vi "Update Method Event Unbundlers.vi"(8 "error in (no error)":errorcluster, 11 "VI ref in":refnum<vi>) -> (0 "error out":errorcluster, 2 "RPC Method Name":string, 3 "VI ref out":refnum<vi>)   [LabVIEW 2019, in "gRPC Scripting Tools.lvlib"]
uses:
  gRPC Scripting Tools.lvlib
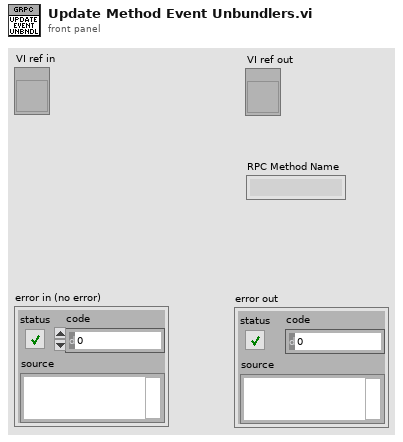
[diagram p1: front panel]
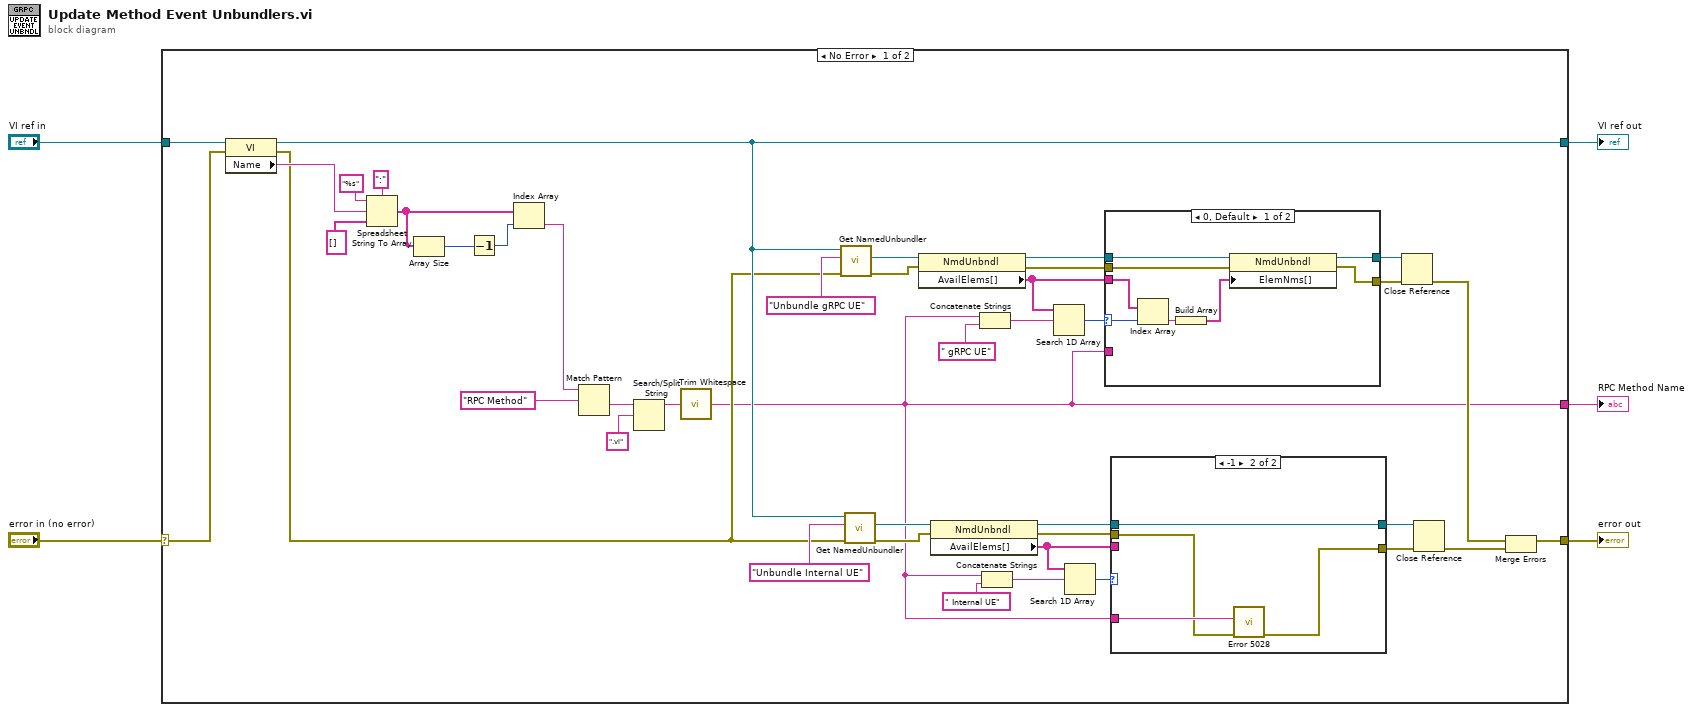
[diagram p0: block diagram]
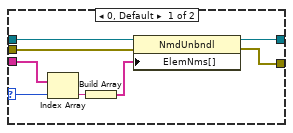
[diagram p2: hidden frame]
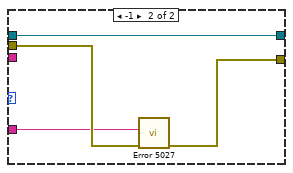
[diagram p3: hidden frame]
diagram:
  n1 = case shown="No Error" "error in (no error)" {
    selector: "error in (no error)" -> [w18 w73]
    tunnel: [w47 w73] -> w5
    tunnel: "VI ref in" -> [w29 w72]
    tunnel: [w28 w72] -> w2
    tunnel: [w6 _] -> w1
    frame No Error {
      n2 = property class="VI"(reference=w29, error in=w18) -> (reference out=w28:refnum<vi>, error out=w17:errorcluster, "Name"=w26:string)
      n3 = Spreadsheet String To Array(delimiter (Tab)=":", format string="%s", spreadsheet string=w26, array type (2D Dbl)=string[] []) -> (array=w21:string[])
      n4 = Array Size(array=w21) -> (size(s)=w23:i32)
      n5 = Decrement(x=w23) -> (x-1=w22:i32)
      n6 = Index Array(array=w21, index=w22) -> (element=w20:string)
      n7 = Match Pattern(string=w20, regular expression="RPC Method") -> (after substring=w16:string)  [unwired: 1 in, 3 out]
      n8 = Search/Split String(string=w16, search string/char (-)=".vi" ("regular expression")) -> (substring before match=w15:string)  [unwired: 1 in, 2 out]
      n9 = call <vilib>:"Trim Whitespace.vi"("string"=w15) -> ("trimmed string"=w6:string)  [unwired: 1 in]
      n10 = call "Get NamedUnbundler.vi"("error in (no error)"=w17, "Label"="Unbundle gRPC UE" ("name/order"), "Owner VI in"=w28) -> ("error out"=w43:errorcluster, "NamedUnbundler ref out"=w31:refnum<vi>)  [unwired: 5 in, 2 out]
      n11 = call "Get NamedUnbundler.vi"("error in (no error)"=w17, "Label"="Unbundle Internal UE" ("name/order"), "Owner VI in"=w28) -> ("error out"=w44:errorcluster, "NamedUnbundler ref out"=w38:refnum<vi>)  [unwired: 5 in, 2 out]
      n12 = property class="NmdUnbndl"(reference=w31, error in=w43) -> (reference out=w35:refnum<vi>, error out=w36:errorcluster, "AvailElems[]"=w34:string[])
      n13 = property class="NmdUnbndl"(reference=w38, error in=w44) -> (reference out=w12:refnum<vi>, error out=w7:errorcluster, "AvailElems[]"=w8:string[])
      n14 = Concatenate Strings(w6, " gRPC UE" ("string")) -> (w33:string)
      n15 = Concatenate Strings(w6, " Internal UE" ("string")) -> (w40:string)
      n16 = Search 1D Array(1D array=w34, element=w33) -> (index of element=w13:i32)  [unwired: 1 in]
      n17 = Search 1D Array(1D array=w8, element=w40) -> (index of element=w11:i32)  [unwired: 1 in]
      n18 = case shown="0, Default" w13 {
        selector: w13 -> [w60 _]
        tunnel: [w67 w71] -> w42
        tunnel: [w66 w69] -> w41
        tunnel: w36 -> [w65 w70]
        tunnel: w35 -> [w62 w71]
        tunnel: w34 -> [w61 _]
        tunnel: w6 -> [_ w68]
        frame 0, Default {
          n19 = Index Array(array=w61, index=w60) -> (element=w63:string)
          n20 = Build Array(w63) -> (w64:string[])
          n21 = property class="NmdUnbndl"(reference=w62, error in=w65, "ElemNms[]"=w64) -> (reference out=w67:refnum<vi>, error out=w66:errorcluster)
        }
        frame -1 {
          n22 = call "Error 5027.vi"("error in (no error)"=w70, "Method Name"=w68) -> ("error out"=w69:errorcluster)  [unwired: 9 in]
        }
      }
      n23 = case shown="-1" w11 {
        selector: w11 -> [w48 _]
        tunnel: [w55 w59] -> w9
        tunnel: [w54 w56] -> w10
        tunnel: w7 -> [w53 w57]
        tunnel: w12 -> [w50 w59]
        tunnel: w8 -> [w49 _]
        tunnel: w6 -> [_ w58]
        frame 0, Default {
          n24 = Index Array(array=w49, index=w48) -> (element=w51:string)
          n25 = Build Array(w51) -> (w52:string[])
          n26 = property class="NmdUnbndl"(reference=w50, error in=w53, "ElemNms[]"=w52) -> (reference out=w55:refnum<vi>, error out=w54:errorcluster)
        }
        frame -1 {
          n27 = call "Error 5028.vi"("error in (no error)"=w57, "Method Name"=w58) -> ("error out"=w56:errorcluster)  [unwired: 9 in]
        }
      }
      n28 = Close Reference(reference=w42, error in (no error)=w41) -> (error out=w45:errorcluster)
      n29 = Close Reference(reference=w9, error in (no error)=w10) -> (error out=w46:errorcluster)
      n30 = Merge Errors(w45, w46) -> (w47:errorcluster)
    }
    frame Error {
    }
  }
  "error out" <- w5
  "VI ref out" <- w2
  "RPC Method Name" <- w1
